vi "omni drive teleop.vi"(0 "Drive RefNum":T3={"DevStatus"={"status"=FALSE, "code"=0, "source"=""}, "Motors[]"=[], "Square Inputs"=FALSE, "Max Output"=1.0}, 1 "X Axis":dbl, 2 "Y Axis":dbl, 3 "Z Axis":dbl, 4 "Drive Mode":T1, 5 "Center Motor":T4={"DeviceStatus"={"status"=FALSE, "code"=0, "source"=""}, "Type"=enum."PWM", "PWM"={"Controller"=enum."Controller 1", "PWM Channel"=enum."Invalid", "DeadBand"={"Name"="", "maxPositivePwm"=0, "minPositivePwm"=0, "centerPwm"=0, "maxNegativePwm"=0, "minNegativePwm"=0, "angularRange"=0}}, "CAN"={"Device Number"=0, "Control Mode"=enum."Percent VBus", "Semaphore"=refnum, "Max Vout"=12.0, "TalonSRX Control Mode"=enum."Percent VBus"}, "Invert"=FALSE, "TransformRef"=refnum, "InvTransformRef"=refnum}) -> ()   [LabVIEW 2014]
uses:
  typedefs/drive mode.ctl
  <vilib>/Rock Robotics/WPI/RobotDrive/WPI_RobotDriveDevRef.ctl
  <vilib>/Rock Robotics/WPI/MotorControl/WPI_MotorControlDeviceRef.ctl
  <vilib>/Rock Robotics/WPI/MotorControl/WPI_MotorControlType.ctl
  <vilib>/Rock Robotics/SystemInterfaces/Typedef/FPGA_TypedefDigitalModule.ctl
  <vilib>/Rock Robotics/SystemInterfaces/DIO/FPGA_DIOPWMChannel.ctl
  <vilib>/Rock Robotics/WPI/PWM/WPI_PWMDeadband.ctl
  <vilib>/Rock Robotics/WPI/CAN/Jaguar/SubVIs/WPI_CANJaguar_ControlMode.ctl
  <vilib>/Rock Robotics/WPI/CAN/TalonSRX/WPI_CANTalonSRX_APIControlMode.ctl
  <vilib>/Rock Robotics/WPI/PWM/WPI_PWMTransform_ConPane.ctl
  global variables/devrefs.vi
  <vilib>/addons/control/pid/pid.llb/PID (DBL).vi
  <vilib>/Rock Robotics/WPI/RobotDrive/WPI_RobotDriveArcadeDrive_Standard(NoSaturation).vi
  global variables/dashboard data.vi
  <vilib>/addons/control/pid/NI_PID_pid.lvlib
panel:
  in  "Omni-Drive Tab Control":enum32{"Drive I/O", "PID", "Motor Controls"}(tab)
  in  "PID Gains":T2={"proportional gain (Kc)"=0.003, "integral time (Ti, min)"=0.0012, "derivative time (Td, min)"=0.001} {"derivative time (Td, min)" step=0.0001 format="%.5f"; "integral time (Ti, min)" step=0.0001 format="%.5f"; "proportional gain (Kc)" step=0.0001 format="%.5f"}
  out "Gyro Temp °C":dbl
  out "Gyro Temp °F":dbl
  out "Setpoint Angle":dbl format="%#_6g°"
  out "Current Angle":dbl format="%#_g°"
  out "PID & Gyro Waveform Chart":cluster{"Angle":dbl, "output":dbl}(graph)
  out "Angular Rate":dbl
  # "Drive the Robot in Either Arcade Style or H-Drive Style"
  # "VI Inputs"
  # "OKish values rev1\nP: 0.00040\nI: 0.00100\nD: 0.00000\n\nPretty Good values\nP: 0.02\nI: 0.005\nD: 0.001\n\nBetter values?\nP: 0.0025\nI: 0.002\nD: 0.001"
  # "Thats a type def so you can't change it to the system\ncontrol otherwise it will no longer by linked to the typedef,\nand you can't re-link it"
  # "Temporary"
  # "Does this empty space make you feel uncomfortable?"
  # "Yes."
  # "I'm glad you feel that way."
  # "Note: Current Angle only updated in H-Drive, \nSetpoint updated in Arcade"
  # "°/sec"
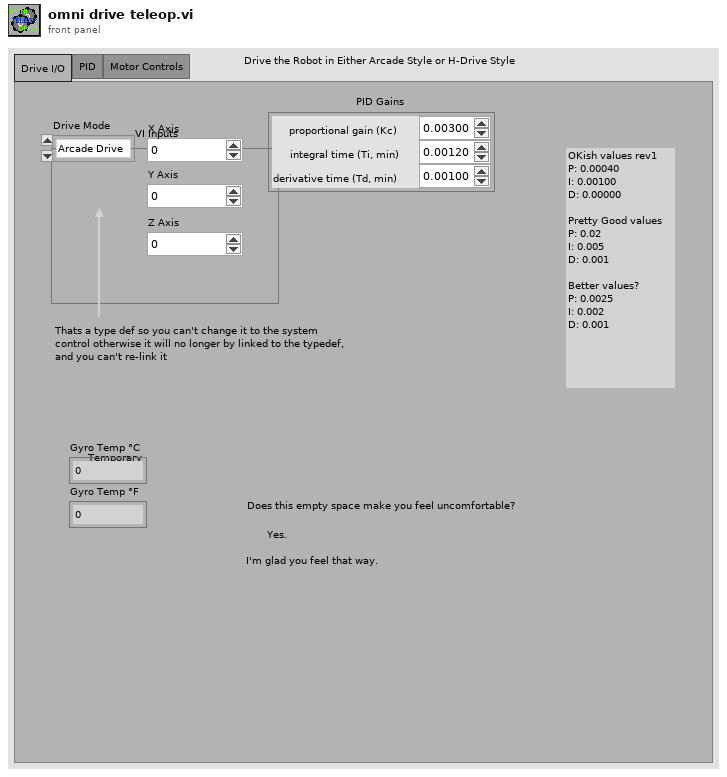
[diagram p1: front panel]
types:
  T1 = typedef "drive mode.ctl" = enum16{"Arcade Drive", "H-Drive", "H-Drive PID"}
  T2 = cluster{"proportional gain (Kc)":dbl, "integral time (Ti, min)":dbl, "derivative time (Td, min)":dbl}
  T3 = typedef "WPI_RobotDriveDevRef.ctl" = cluster{"DevStatus":errorcluster, "Motors[]":T4[], "Square Inputs":bool, "Max Output":dbl}
  T4 = typedef "WPI_MotorControlDeviceRef.ctl" = cluster{"DeviceStatus":errorcluster, "Type":T5, "PWM":cluster{"Controller":T6, "PWM Channel":T7, "DeadBand":T8}, "CAN":cluster{"Device Number":u8, "Control Mode":T9, "Semaphore":T10, "Max Vout":dbl, "TalonSRX Control Mode":T11}, "Invert":bool, "TransformRef":T12, "InvTransformRef":T12}
  T5 = typedef "WPI_MotorControlType.ctl" = enum16{"PWM", "CAN", "CANTalonSRX"}
  T6 = typedef "FPGA_TypedefDigitalModule.ctl" = enum16{"Controller 1"}
  T7 = typedef "FPGA_DIOPWMChannel.ctl" = enum8{"PWM 0", "PWM 1", "PWM 2", "PWM 3", "PWM 4", "PWM 5", "PWM 6", "PWM 7", "PWM 8", "PWM 9", "PWM MXP 0", "PWM MXP 1", "PWM MXP 2", "PWM MXP 3", "PWM MXP 4", "PWM MXP 5", "PWM MXP 6", "PWM MXP 7", "PWM MXP 8", "PWM MXP 9", "Invalid"}
  T8 = typedef "WPI_PWMDeadband.ctl" = cluster{"Name":string, "maxPositivePwm":i32, "minPositivePwm":i32, "centerPwm":i32, "maxNegativePwm":i32, "minNegativePwm":i32, "angularRange":u16}
  T9 = typedef "WPI_CANJaguar_ControlMode.ctl" = enum8{"Percent VBus", "Current", "Speed", "Position", "Voltage"}
  T10 = typedef "Semaphore RefNum" = refnum<k1>
  T11 = typedef "WPI_CANTalonSRX_APIControlMode.ctl" = enum8{"Percent VBus", "Speed", "Position", "Slave", "Unchanged / Invalid"}
  T12 = typedef "WPI_PWMTransform_ConPane.ctl" = refnum<vi>
  T13 = typedef "WPI_GyroDevRef.ctl" = cluster{"DevStatus":errorcluster, "Analog Module":T14, "Analog Channel":T15, "Offset":dbl, "Gain (VoltsPerDegree/Second)":dbl}
  T14 = typedef "FPGA_TypedefAnalogModule.ctl" = enum16{"Controller 1"}
  T15 = typedef "FPGA_AIChannel.ctl" = enum8{"AI 0", "AI 1", "AI 2", "AI 3", "AI MXP 0", "AI MXP 1", "AI MXP 2", "AI MXP 3", "Invalid"}
  T16 = typedef "WPI_EncoderDevRef.ctl" = cluster{"DevStatus":errorcluster, "EncoderIndex":T17, "CounterIndex":T18, "DistancePerCount":dbl, "Decoding Type":T19}
  T17 = typedef "FPGA_EncoderIdx.ctl" = enum8{"Enc 0", "Enc 1", "Enc 2", "Enc 3", "Enc 4", "Enc 5", "Enc 6", "Enc 7", "Invalid"}
  T18 = typedef "FPGA_CounterCtrSystemIndex.ctl" = enum8{"Ctr 0", "Ctr 1", "Ctr 2", "Ctr 3", "Ctr 4", "Ctr 5", "Ctr 6", "Ctr 7", "Invalid"}
  T19 = typedef "WPI_EncoderType.ctl" = enum16{"1x", "2x", "4x"}
  T20 = typedef "WPI_AnalogChannelDevRef.ctl" = cluster{"DevStatus":errorcluster, "Controller":T14, "Analog Channel":T15}
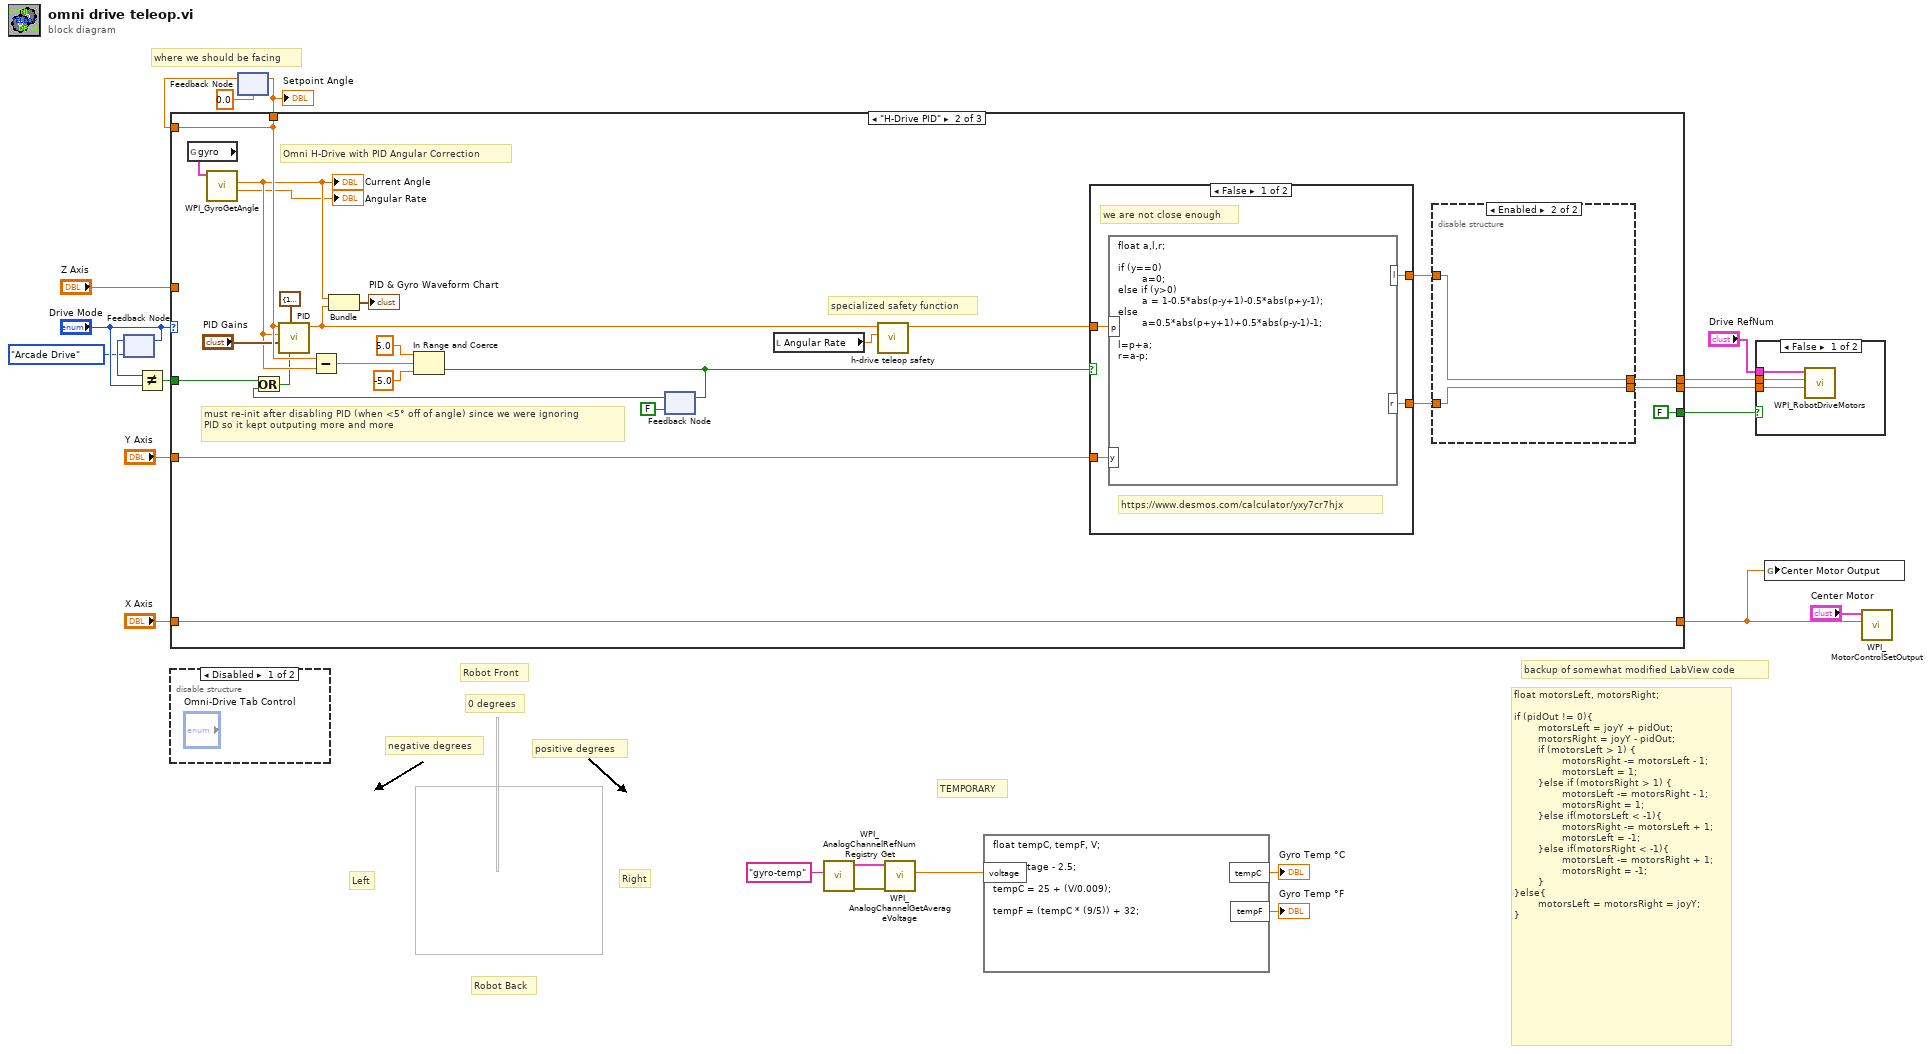
[diagram p0: block diagram]
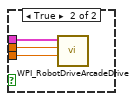
[diagram p3: hidden frame]
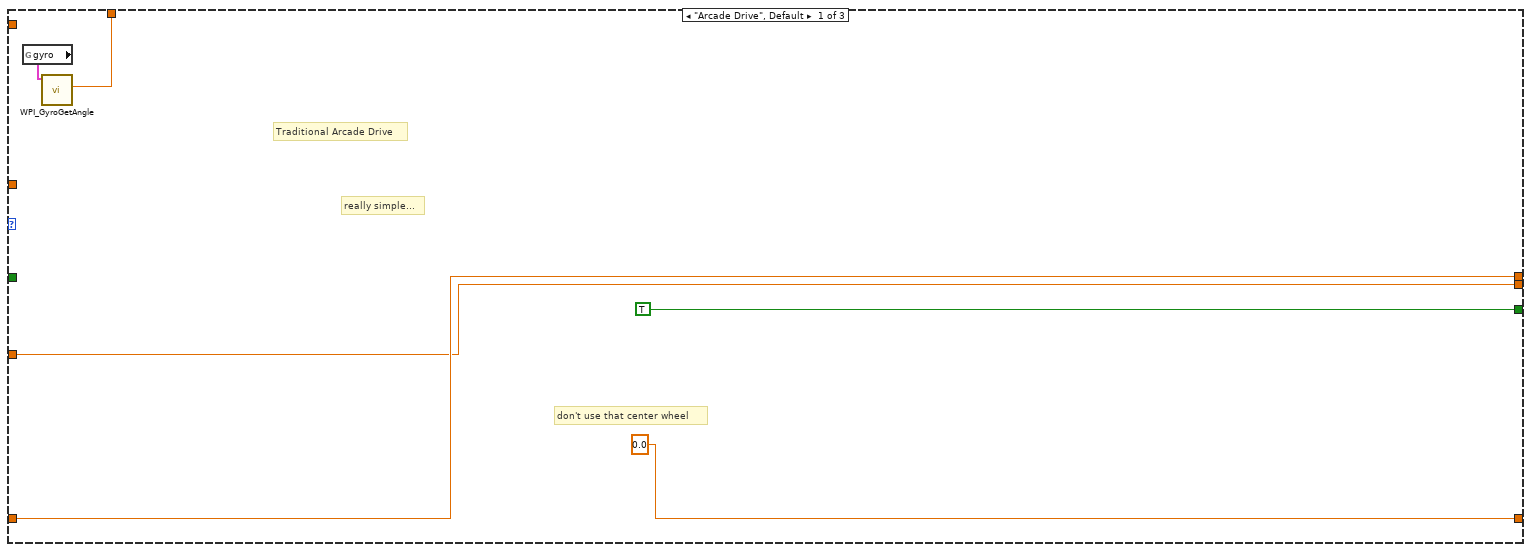
[diagram p4: hidden frame]
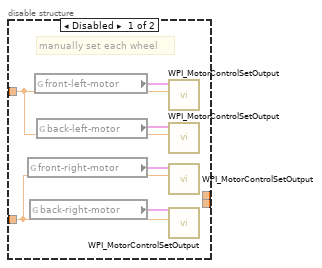
[diagram p5: hidden frame]
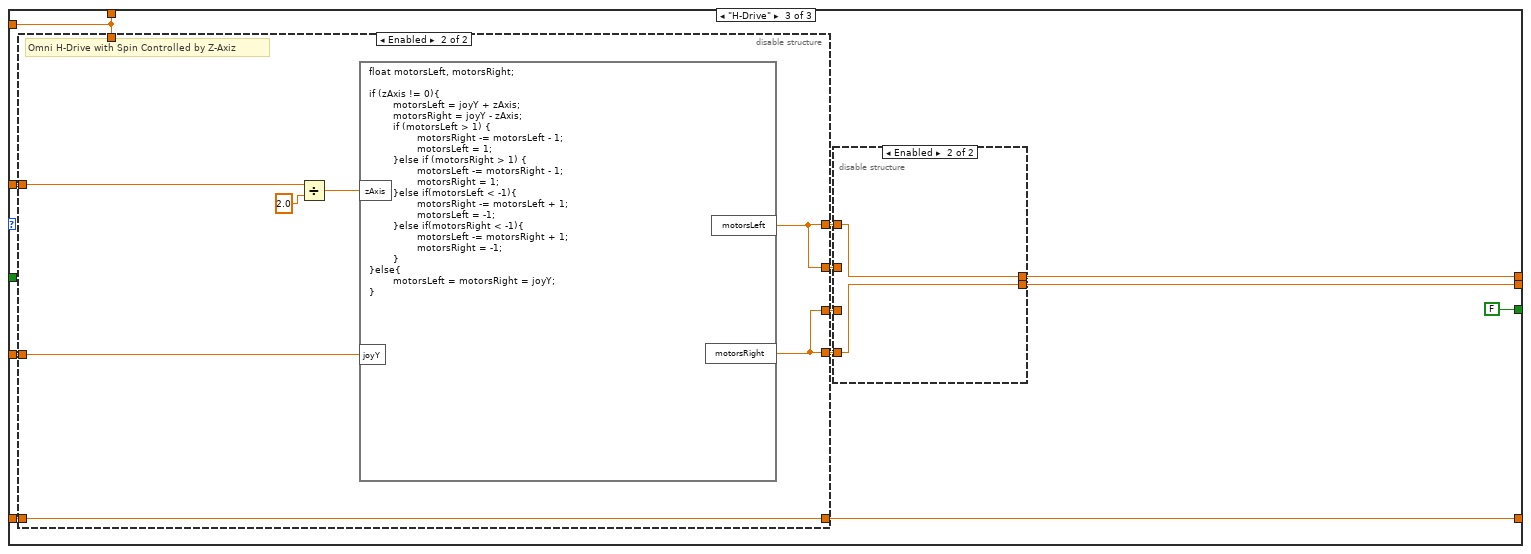
[diagram p7: hidden frame]
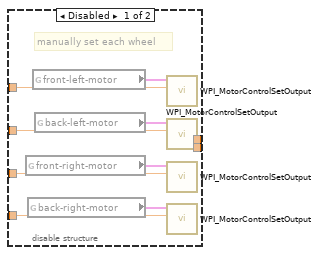
[diagram p8: hidden frame]
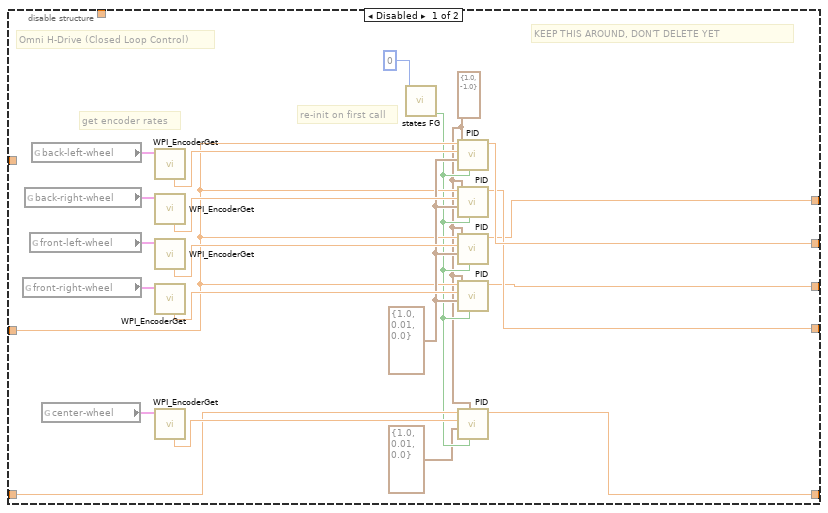
[diagram p9: hidden frame]
diagram:
  # "TEMPORARY"
  # "backup of somewhat modified LabView code"
  # "float motorsLeft, motorsRight;\n\nif (pidOut != 0){\n        motorsLeft = joyY + pidOut;\n        motorsRight = joyY - pidOut;\n        if (motorsLeft > 1) {\n                motorsRight -= motorsLeft - 1;\n                motorsLeft = 1;\n        }else if (motorsRight > 1) {\n                motorsLeft -= motorsRight - 1;\n                motorsRight = 1;\n        }else if(motorsLeft < -1){\n                motorsRight -= motorsLeft + 1;\n                motorsLeft = -1;\n        }else if(motorsRight < -1){\n                motorsLeft -= motorsRight + 1;\n                motorsRight = -1;\n        }\n}else{\n        motorsLeft = motorsRight = joyY;\n}"
  # "Robot Back"
  # "Right"
  # "Left"
  # "negative degrees"
  # "positive degrees"
  # "0 degrees"
  # "Robot Front"
  # "where we should be facing"
  n1 = feedback-in #1("Drive Mode") -> ()
  n2 = feedback #1(drive_mode."Arcade Drive" ("Drive Mode")) -> (w15:T1)
  n3 = Not Equal?(x=w15, y="Drive Mode") -> (x != y?=w13:bool)
  n4 = disable-structure shown="Disabled" {
    frame Disabled {
    }
    frame Enabled {
    }
  }
  n5 = feedback #2(0.0) -> (w11:dbl)
  n6 = case shown="\"H-Drive PID\"" "Drive Mode" {
    tunnel: [0.0 w51 w75] -> w1
    tunnel: [w27 w29 w67] -> w22
    tunnel: [w28 w30 w68] -> w21
    tunnel: "X Axis" -> [w28 w51 w76]
    tunnel: "Y Axis" -> [w27 w52 w77]
    tunnel: [TRUE FALSE FALSE] -> w18
    tunnel: w13 -> [_ w50 _]
    tunnel: [w24 w49 w74] -> w12
    tunnel: w11 -> [_ w49 w74]
    tunnel: "Z Axis" -> [_ _ w69]
    frame "Arcade Drive", Default {
      # "really simple..."
      # "don't use that center wheel"
      # "Traditional Arcade Drive"
      n7 = global read "devrefs.vi" "gyro"() -> (w25:T13)
      n8 = call <vilib>:"WPI_GyroGetAngle.vi"("GyroDevRef"=w25) -> ("Angle"=w24:dbl)  [unwired: 7 in, 3 out]
    }
    frame "H-Drive PID" {
      # "specialized safety function"
      # "must re-init after disabling PID (when <5° off of angle) since we were ignoring\nPID so it kept outputing more and more"
      # "Omni H-Drive with PID Angular Correction"
      n9 = global read "devrefs.vi" "gyro"() -> (w45:T13)
      n10 = call <vilib>:"WPI_GyroGetAngle.vi"("GyroDevRef"=w45) -> ("Angular Rate"=→"Angular Rate":dbl, "Angle"=w42:dbl)  [unwired: 7 in, 2 out]
      "Current Angle" <- w42
      n11 = Subtract(x=w49, y=w42) -> (x-y=w38:dbl)
      n12 = In Range and Coerce(upper limit=5.0, x=w38, lower limit=-5.0 ("upper limit")) -> (In Range?=w41:bool)  [unwired: 1 out]
      n13 = feedback #3(FALSE) -> (w35:bool)
      n14 = Or(x=w50, y=w35) -> (x .or. y?=w40:bool)
      n15 = call-poly <vilib>:"PID.vi"("reinitialize? (F)"=w40, "output range"=cluster{"output high":dbl, "output low":dbl} {"output high"=1.0, "output low"=-1.0}, "PID gains"="PID Gains", "process variable"=w42, "setpoint"=w49) -> ("output"=w33:dbl)  [unwired: 5 in, 1 out]
      n16 = Bundle("Angle"=w42, "output"=w33) -> (→"PID & Gyro Waveform Chart":cluster{"Angle":dbl, "output":dbl})  [unwired: 1 in]
      n17 = feedback-in #3(w41) -> ()
      n18 = local read "Angular Rate"() -> (w31:dbl)
      n19 = call "h-drive teleop safety.vi"("Gyro Angular Rate"=w31, "Input"=w33) -> ("Output"=w32:dbl)  [unwired: 9 in]
      n20 = case shown="False" w41 {
        tunnel: w32 -> [w63 _]
        tunnel: w52 -> [w62 w66]
        tunnel: [w65 w66] -> w47
        tunnel: [w64 w66] -> w48
        frame False {
          # "https://www.desmos.com/calculator/yxy7cr7hjx"
          # "we are not close enough"
          n21 = formula code="float a,l,r;\n\nif (y==0) \n        a=0;\nelse if (y>0) \n        a = 1-0.5*abs(p-y+1)-0.5*abs(p+y-1);\nelse \n        a=0.5*abs(p+y+1)+0.5*abs(p-y-1)-1;\n\nl=p+a;\nr=a-p;"("p"=w63, "y"=w62) -> ("l"=w64:dbl, "r"=w65:dbl)
        }
        frame True {
          # "close enough... within 5°"
        }
      }
      n22 = disable-structure shown="Enabled" {
        disable-tunnel: w48 -> [w55 w61]
        disable-tunnel: w47 -> [w54 w60]
        disable-tunnel: [_ w61] -> w30
        disable-tunnel: [_ w60] -> w29
        frame Disabled {
          # "manually set each wheel"
          n23 = global read "devrefs.vi" "front-right-motor"() -> (w56:T4)
          n24 = global read "devrefs.vi" "back-right-motor"() -> (w58:T4)
          n25 = global read "devrefs.vi" "front-left-motor"() -> (w57:T4)
          n26 = global read "devrefs.vi" "back-left-motor"() -> (w59:T4)
          n27 = call <vilib>:"WPI_MotorControlSetOutput.vi"("Output"=w55, "MotorControlDevRef"=w57) -> ()  [unwired: 7 in, 3 out]
          n28 = call <vilib>:"WPI_MotorControlSetOutput.vi"("Output"=w55, "MotorControlDevRef"=w59) -> ()  [unwired: 7 in, 3 out]
          n29 = call <vilib>:"WPI_MotorControlSetOutput.vi"("Output"=w54, "MotorControlDevRef"=w56) -> ()  [unwired: 7 in, 3 out]
          n30 = call <vilib>:"WPI_MotorControlSetOutput.vi"("Output"=w54, "MotorControlDevRef"=w58) -> ()  [unwired: 7 in, 3 out]
        }
        frame Enabled {
        }
      }
    }
    frame "H-Drive" {
      n31 = disable-structure shown="Enabled" {
        disable-tunnel: w77 -> [w99 w117]
        disable-tunnel: w76 -> [w97 w116]
        disable-tunnel: [w93 w116] -> w75
        disable-tunnel: w74 -> [_ _]
        disable-tunnel: [w90 w115] -> w73
        disable-tunnel: [w92 w115] -> w72
        disable-tunnel: [w91 w114] -> w70
        disable-tunnel: [w89 w114] -> w71
        disable-tunnel: w69 -> [_ w111]
        frame Disabled {
          w100 = T2 {"proportional gain (Kc)"=1.0, "integral time (Ti, min)"=0.01, "derivative time (Td, min)"=0.0} ("PID gains")
          w95 = cluster{"output high":dbl, "output low":dbl} {"output high"=1.0, "output low"=-1.0} ("output range")
          # "KEEP THIS AROUND, DON'T DELETE YET"
          # "re-init on first call"
          # "get encoder rates"
          # "Omni H-Drive (Closed Loop Control)"
          n32 = global read "devrefs.vi" "front-right-wheel"() -> (w107:T16)
          n33 = global read "devrefs.vi" "back-right-wheel"() -> (w109:T16)
          n34 = global read "devrefs.vi" "front-left-wheel"() -> (w108:T16)
          n35 = global read "devrefs.vi" "back-left-wheel"() -> (w110:T16)
          n36 = global read "devrefs.vi" "center-wheel"() -> (w106:T16)
          n37 = call <vilib>:"WPI_EncoderGet.vi"("EncoderDevRef"=w110) -> ("Rate"=w104:dbl)  [unwired: 5 in, 5 out]
          n38 = call <vilib>:"WPI_EncoderGet.vi"("EncoderDevRef"=w109) -> ("Rate"=w103:dbl)  [unwired: 5 in, 5 out]
          n39 = call <vilib>:"WPI_EncoderGet.vi"("EncoderDevRef"=w108) -> ("Rate"=w102:dbl)  [unwired: 5 in, 5 out]
          n40 = call <vilib>:"WPI_EncoderGet.vi"("EncoderDevRef"=w107) -> ("Rate"=w101:dbl)  [unwired: 5 in, 5 out]
          n41 = call <vilib>:"WPI_EncoderGet.vi"("EncoderDevRef"=w106) -> ("Rate"=w98:dbl)  [unwired: 5 in, 5 out]
          n42 = call "states FG.vi"("Loop ID"=0) -> ("first call?"=w96:bool)  [unwired: 7 in, 3 out]
          n43 = call-poly <vilib>:"PID.vi"("reinitialize? (F)"=w96, "output range"=w95, "PID gains"=w100, "process variable"=w104, "setpoint"=w99) -> ("output"=w92:dbl)  [unwired: 5 in, 1 out]
          n44 = call-poly <vilib>:"PID.vi"("reinitialize? (F)"=w96, "output range"=w95, "PID gains"=w100, "process variable"=w103, "setpoint"=w99) -> ("output"=w91:dbl)  [unwired: 5 in, 1 out]
          n45 = call-poly <vilib>:"PID.vi"("reinitialize? (F)"=w96, "output range"=w95, "PID gains"=w100, "process variable"=w102, "setpoint"=w99) -> ("output"=w90:dbl)  [unwired: 5 in, 1 out]
          n46 = call-poly <vilib>:"PID.vi"("reinitialize? (F)"=w96, "output range"=w95, "PID gains"=w100, "process variable"=w101, "setpoint"=w99) -> ("output"=w89:dbl)  [unwired: 5 in, 1 out]
          n47 = call-poly <vilib>:"PID.vi"("reinitialize? (F)"=w96, "output range"=w95, "PID gains"=T2 {"proportional gain (Kc)"=1.0, "integral time (Ti, min)"=0.01, "derivative time (Td, min)"=0.0}, "process variable"=w98, "setpoint"=w97) -> ("output"=w93:dbl)  [unwired: 5 in, 1 out]
        }
        frame Enabled {
          # "Omni H-Drive with Spin Controlled by Z-Axiz"
          n48 = Divide(x=w111, y=2.0) -> (x/y=w112:dbl)
          n49 = formula code="float motorsLeft, motorsRight;\n\nif (zAxis != 0){\n        motorsLeft = joyY + zAxis;\n        motorsRight = joyY - zAxis;\n        if (motorsLeft > 1) {\n                motorsRight -= motorsLeft - 1;\n                motorsLeft = 1;\n        }else if (motorsRight > 1) {\n                motorsLeft -= motorsRight - 1;\n                motorsRight = 1;\n        }else if(motorsLeft < -1){\n                motorsRight -= motorsLeft + 1;\n                motorsLeft = -1;\n        }else if(motorsRight < -1){\n                motorsLeft -= motorsRight + 1;\n                motorsRight = -1;\n        }\n}else{\n        motorsLeft = motorsRight = joyY;\n}"("zAxis"=w112, "joyY"=w117) -> ("motorsLeft"=w115:dbl, "motorsRight"=w114:dbl)
        }
      }
      n50 = disable-structure shown="Enabled" {
        disable-tunnel: w73 -> [w82 w88]
        disable-tunnel: w72 -> [w81 _]
        disable-tunnel: w71 -> [w80 _]
        disable-tunnel: w70 -> [w79 w87]
        disable-tunnel: [_ w88] -> w68
        disable-tunnel: [_ w87] -> w67
        frame Disabled {
          # "manually set each wheel"
          n51 = global read "devrefs.vi" "front-right-motor"() -> (w83:T4)
          n52 = global read "devrefs.vi" "back-right-motor"() -> (w85:T4)
          n53 = global read "devrefs.vi" "front-left-motor"() -> (w84:T4)
          n54 = global read "devrefs.vi" "back-left-motor"() -> (w86:T4)
          n55 = call <vilib>:"WPI_MotorControlSetOutput.vi"("Output"=w82, "MotorControlDevRef"=w84) -> ()  [unwired: 7 in, 3 out]
          n56 = call <vilib>:"WPI_MotorControlSetOutput.vi"("Output"=w81, "MotorControlDevRef"=w86) -> ()  [unwired: 7 in, 3 out]
          n57 = call <vilib>:"WPI_MotorControlSetOutput.vi"("Output"=w80, "MotorControlDevRef"=w83) -> ()  [unwired: 7 in, 3 out]
          n58 = call <vilib>:"WPI_MotorControlSetOutput.vi"("Output"=w79, "MotorControlDevRef"=w85) -> ()  [unwired: 7 in, 3 out]
        }
        frame Enabled {
        }
      }
    }
  }
  "Setpoint Angle" <- w12
  n59 = feedback-in #2(w12) -> ()
  n60 = call <vilib>:"WPI_AnalogChannelRefNum Registry Get.vi"("refnum name"="gyro-temp") -> ("error out"=w7:errorcluster, "AIDeviceRef"=w6:T20)  [unwired: 9 in]
  n61 = call <vilib>:"WPI_AnalogChannelGetAverageVoltage.vi"("error in (no error)"=w7, "AIDeviceRef"=w6) -> ("Voltage"=w4:dbl)  [unwired: 7 in, 2 out]
  n62 = formula code="float tempC, tempF, V;\n\nV = voltage - 2.5;\n\ntempC = 25 + (V/0.009);\n\ntempF = (tempC * (9/5)) + 32;"("voltage"=w4) -> ("tempC"=→"Gyro Temp °C":dbl, "tempF"=→"Gyro Temp °F":dbl)
  n63 = case shown="False" w18 {
    tunnel: "Drive RefNum" -> [w120 w123]
    tunnel: w22 -> [w118 w122]
    tunnel: w21 -> [w119 w121]
    frame False {
      n64 = call <vilib>:"WPI_RobotDriveMotors.vi"("RightSpeed"=w118, "LeftSpeed"=w119, "RobotDriveDevRef"=w120) -> ()  [unwired: 6 in, 3 out]
    }
    frame True {
      n65 = call-poly <vilib>:"WPI_RobotDriveArcadeDrive.vi"("Y axis value"=w122, "X axis value"=w121, "RobotDriveDevRef"=w123) -> ()  [unwired: 6 in, 3 out]
    }
  }
  n66 = global write "dashboard data.vi" "Center Motor Output"(w1) -> ()
  n67 = call <vilib>:"WPI_MotorControlSetOutput.vi"("Output"=w1, "MotorControlDevRef"="Center Motor") -> ()  [unwired: 7 in, 3 out]
